vi "resetPressures_topLvl.vi"(8 "error in":errorcluster, 11 "Pressure box control in":T1={"Pressure box COM"="", "pressure box type"=enum."Neuromatics", "High pos pressure (mBar)"=200.0, "Low pos pressure (mBar)"=80.0, "Vacuum pressure (mBar)"=-40.0, "calibration"=enum."PA_vacPump"}) -> (0 "error out":errorcluster, 3 "Pressure box control out":T1={"Pressure box COM"="", "pressure box type"=enum."Neuromatics", "High pos pressure (mBar)"=200.0, "Low pos pressure (mBar)"=80.0, "Vacuum pressure (mBar)"=-40.0, "calibration"=enum."PA_vacPump"})   [LabVIEW 2015]
uses:
  controls/pressure_box_type.ctl
  controls/pressure_box_control.ctl
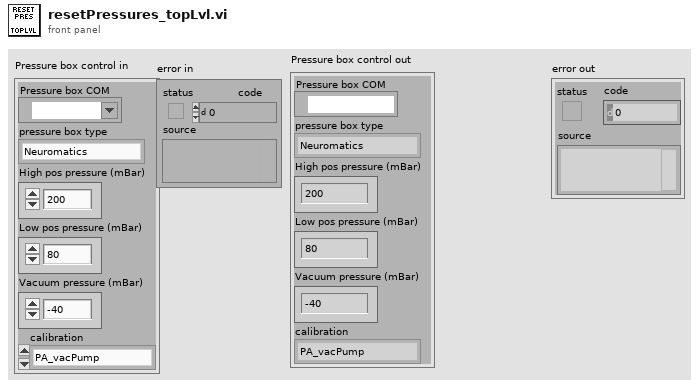
[diagram p1: front panel]
types:
  T1 = typedef "pressure_box_control.ctl" = cluster{"Pressure box COM":refnum<visa-resource-name>, "pressure box type":T2, "High pos pressure (mBar)":dbl, "Low pos pressure (mBar)":dbl, "Vacuum pressure (mBar)":dbl, "calibration":enum16{"PA_vacPump", "PA_venturi", "Neuromatics", "ilyaRig", "mightenRig"}}
  T2 = typedef "pressure_box_type.ctl" = enum16{"Neuromatics", "ProportionAir", "Demo box", "N-ProportionAir"}
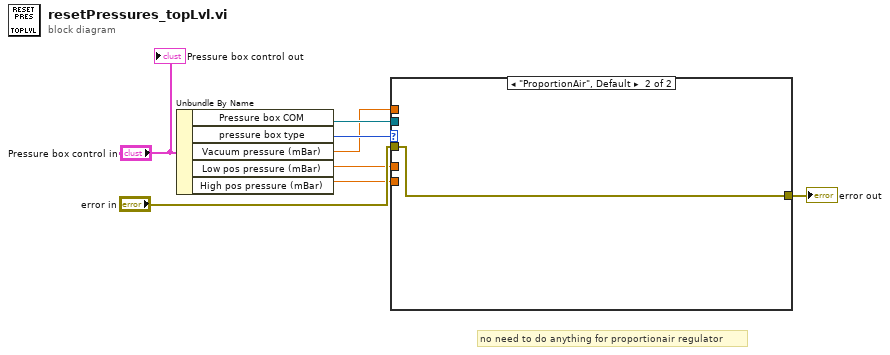
[diagram p0: block diagram]
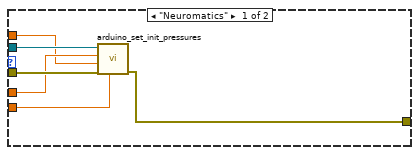
[diagram p2: hidden frame]
diagram:
  # "no need to do anything for proportionair regulator"
  n1 = Unbundle By Name("Pressure box control in") -> ("Pressure box COM"=w6:refnum<visa-resource-name>, "pressure box type"=w7:T2, "Vacuum pressure (mBar)"=w3:dbl, "Low pos pressure (mBar)"=w4:dbl, "High pos pressure (mBar)"=w2:dbl)
  n2 = case shown="\"ProportionAir\", Default" w7 {
    tunnel: w6 -> [w14 _]
    tunnel: "error in" -> [w13 w15]
    tunnel: w4 -> [w12 _]
    tunnel: w3 -> [w11 _]
    tunnel: w2 -> [w10 _]
    tunnel: [w9 w15] -> w1
    frame "Neuromatics" {
      n3 = call "arduino_set_init_pressures.vi"("High P"=w10, "error in"=w13, "Suction"=w11, "Low P"=w12, "Pressure Box COM in"=w14) -> ("error out"=w9:errorcluster)  [unwired: 5 in, 1 out]
    }
    frame "ProportionAir", Default {
    }
  }
  "error out" <- w1
  "Pressure box control out" <- "Pressure box control in"
